vi "dvp Vi Get Anti Flick.vi"(10 "pAntiFlick":u32(ring) items=["ANTIFLICK_DISABLE", "ANTIFLICK_50HZ", "ANTIFLICK_60HZ"], 11 "handle":u32) -> (2 "pAntiFlick out":u32(ring) items=["ANTIFLICK_DISABLE", "ANTIFLICK_50HZ", "ANTIFLICK_60HZ"], 3 "function return":u32(ring))   [LabVIEW 2018, in "LabViewDVPCamera.lvlib"]
doc: "LabviewDvp2Api dvpStatus dvpViGetAntiFlick(dvpHandle handle, dvpAntiFlick *pAntiFlick);"
uses:
  LabViewDVPCamera.lvlib
  LabViewDVPCamera/LabViewDVPCamera.dll
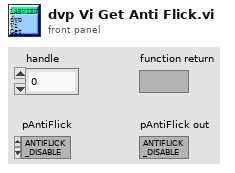
[diagram p1: front panel]
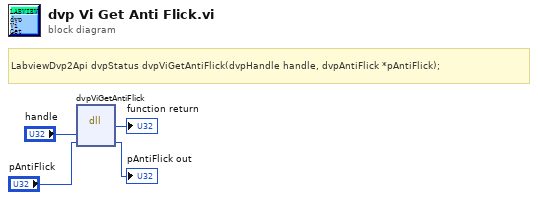
[diagram p0: block diagram]
diagram:
  # "LabviewDvp2Api dvpStatus dvpViGetAntiFlick(dvpHandle handle, dvpAntiFlick *pAntiFlick);"
  n1 = dll-call lib="C:/Program Files (x86)/DVP2 Labview cn 64/Sample/LabViewDVPCamera/LabViewDVPCamera.*" fn="dvpViGetAntiFlick"("handle"="handle", "pAntiFlick"="pAntiFlick") -> (→"function return":u32, "pAntiFlick"=→"pAntiFlick out":u32)  [unwired: 4 in, 2 out]
